vi "Detailed Logging.vi"(8 "error in":errorcluster, 11 "DIG_IO in":refnum<class "DIG_IO.lvclass">) -> (0 "error out":errorcluster, 2 "Detailed Record":waveform(i16)[](array[waveform]), 3 "DIG_IO out":refnum<class "DIG_IO.lvclass">)   [LabVIEW 2019, in "DIG_IO.lvlib" / "DIG_IO.lvclass"]
uses:
  Library/DIG_IO.lvclass
  C:/Users/Public/Documents/Development/builds/Instruments/Instruments.lvlibp/Library/Instruments.lvclass
  Library/DIG_IO.lvclass/DIG_IO.ctl
  Accessors/Read Banks.vi
  Accessors/Read Channel Names.vi
  builds/Instruments/Instruments.lvlibp/Accessors/Read dt.vi
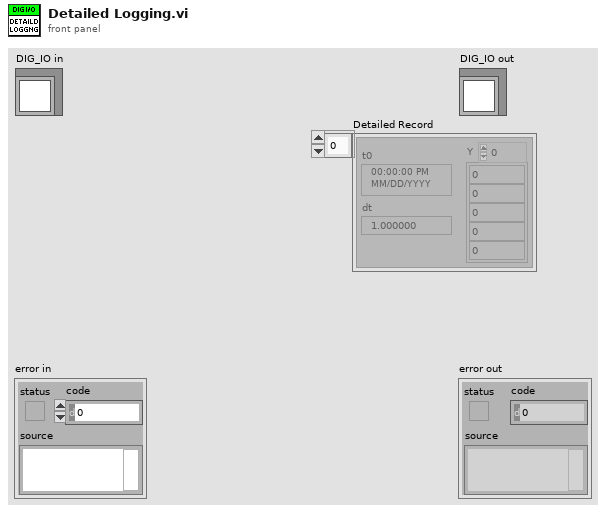
[diagram p1: front panel]
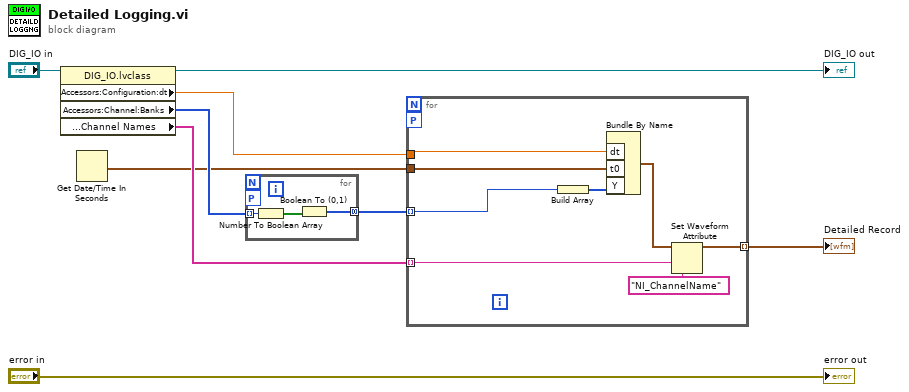
[diagram p0: block diagram]
diagram:
  n1 = property class="DIG_IO.lvclass"(reference="DIG_IO in") -> (reference out=→"DIG_IO out":refnum<class "DIG_IO.lvclass">, "Accessors:Configuration:dt"=w5:dbl, "Accessors:Channel:Banks"=w7:u8[], "Accessors:Channel:Channel Names"=w9:string[])  [unwired: 1 in, 1 out]
  n2 = Get Date/Time In Seconds() -> (seconds since 1Jan1904=w6:timestamp)
  n3 = for {
    tunnel: w7 -> [w12] mode=indexing
    tunnel: [w10] -> w8 mode=concatenating
    workers-P: _ -> [_]
    n4 = Number To Boolean Array(number=w12) -> (Boolean array=w11:bool[])
    n5 = Boolean To (0,1)(Boolean=w11) -> (0, 1=w10:i16[])
  }
  n6 = for {
    tunnel: w8 -> [w20] mode=indexing
    tunnel: [w18] -> w1 mode=indexing
    tunnel: w6 -> [w14]
    workers-P: _ -> [_]
    tunnel: w5 -> [w16]
    tunnel: w9 -> [w13] mode=indexing
    n7 = Build Array(w20) -> (w15:i16[])
    n8 = Bundle By Name("dt"=w16, "t0"=w14, "Y"=w15) -> (w19:waveform(i16))  [unwired: 1 in]
    n9 = Set Waveform Attribute(5:w13, 6:"NI_ChannelName" ("name"), 7:w19) -> (3:w18:waveform(i16))  [unwired: 1 in, 2 out]
  }
  "Detailed Record" <- w1
  "error out" <- "error in"
